vi "victory march sub vi (adjusted).vi"(11 "BrickReference in":T1) -> (3 "BrickReference out":T1)   [LabVIEW 2016]
uses:
  <vilib>/NXT/Subs/LVHSConnector.ctl
  <vilib>/NXT/LegoClasses/BrickReference/BrickReference.lvclass
  <vilib>/NXT/Dual Mode Library/Sound/PlayB.vi
  <vilib>/NXT/Dual Mode Library/Sound/PlayAsharp.vi
  <vilib>/NXT/Dual Mode Library/Sound/PlayC.vi
  <vilib>/NXT/Dual Mode Library/Sound/PlayD.vi
  <vilib>/NXT/Dual Mode Library/Sound/PlayE.vi
  <vilib>/NXT/Dual Mode Library/Sound/PlayG.vi
  <vilib>/NXT/Dual Mode Library/Sound/PlayFsharp.vi
  <vilib>/NXT/Dual Mode Library/Sound/PlayA.vi
  <vilib>/NXT/Dual Mode Library/Waits/Wait_Num.vi
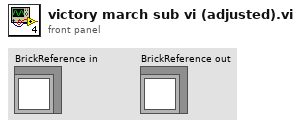
[diagram p1: front panel]
types:
  T1 = typedef "LVHSConnector.ctl" = refnum<class "BrickReference.lvclass">
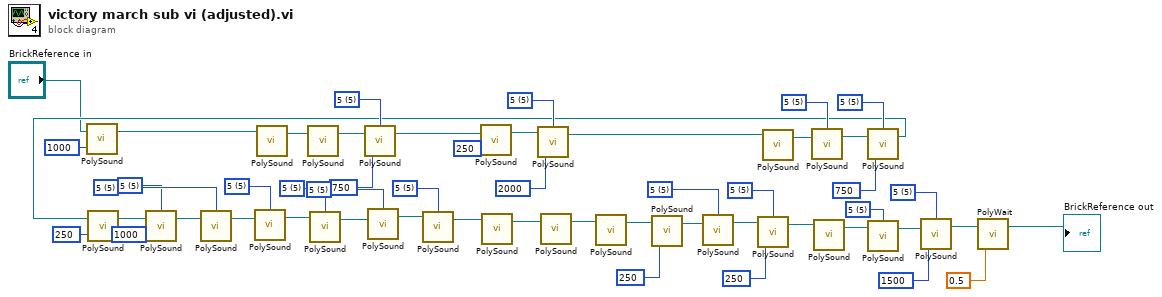
[diagram p0: block diagram]
diagram:
  w51 = u16 5 items=["3"=3, "4"=4, "5"=5, "6"=6, "7"=7] ("Octave")
  w50 = u16 5 items=["3"=3, "4"=4, "5"=5, "6"=6, "7"=7] ("Octave")
  w49 = u16 5 items=["3"=3, "4"=4, "5"=5, "6"=6, "7"=7] ("Octave")
  w48 = u16 5 items=["3"=3, "4"=4, "5"=5, "6"=6, "7"=7] ("Octave")
  w44 = u16 5 items=["3"=3, "4"=4, "5"=5, "6"=6, "7"=7] ("Octave")
  w43 = u16 5 items=["3"=3, "4"=4, "5"=5, "6"=6, "7"=7] ("Octave")
  w42 = u16 5 items=["3"=3, "4"=4, "5"=5, "6"=6, "7"=7] ("Octave")
  w41 = u16 5 items=["3"=3, "4"=4, "5"=5, "6"=6, "7"=7] ("Octave")
  w40 = u16 5 items=["3"=3, "4"=4, "5"=5, "6"=6, "7"=7] ("Octave")
  w36 = u16 5 items=["3"=3, "4"=4, "5"=5, "6"=6, "7"=7] ("Octave")
  w35 = u16 5 items=["3"=3, "4"=4, "5"=5, "6"=6, "7"=7] ("Octave")
  w34 = u16 5 items=["3"=3, "4"=4, "5"=5, "6"=6, "7"=7] ("Octave")
  w33 = u16 5 items=["3"=3, "4"=4, "5"=5, "6"=6, "7"=7] ("Octave")
  w32 = u16 5 items=["3"=3, "4"=4, "5"=5, "6"=6, "7"=7] ("Octave")
  n1 = call-poly <vilib>:"PolySound.vi"("Duration (500 ms)"=u16 1000, "NXT/EV3"="BrickReference in") -> ("NXT/EV3"=w5:T1)  [unwired: 2 in]
  n2 = call-poly <vilib>:"PolySound.vi"("NXT/EV3"=w5) -> ("NXT/EV3"=w6:T1)  [unwired: 3 in]
  n3 = call-poly <vilib>:"PolySound.vi"("NXT/EV3"=w6) -> ("NXT/EV3"=w7:T1)  [unwired: 3 in]
  n4 = call-poly <vilib>:"PolySound.vi"("Duration (500 ms)"=u16 750, "NXT/EV3"=w7, "Octave"=w32) -> ("NXT/EV3"=w4:T1)  [unwired: 1 in]
  n5 = call-poly <vilib>:"PolySound.vi"("Duration (500 ms)"=u16 250, "NXT/EV3"=w4) -> ("NXT/EV3"=w8:T1)  [unwired: 2 in]
  n6 = call-poly <vilib>:"PolySound.vi"("Duration (500 ms)"=u16 2000, "NXT/EV3"=w8, "Octave"=w33) -> ("NXT/EV3"=w3:T1)  [unwired: 1 in]
  n7 = call-poly <vilib>:"PolySound.vi"("NXT/EV3"=w3) -> ("NXT/EV3"=w9:T1)  [unwired: 3 in]
  n8 = call-poly <vilib>:"PolySound.vi"("NXT/EV3"=w9, "Octave"=w34) -> ("NXT/EV3"=w10:T1)  [unwired: 2 in]
  n9 = call-poly <vilib>:"PolySound.vi"("Duration (500 ms)"=u16 750, "NXT/EV3"=w10, "Octave"=w35) -> ("NXT/EV3"=w2:T1)  [unwired: 1 in]
  n10 = call-poly <vilib>:"PolySound.vi"("Duration (500 ms)"=u16 250, "NXT/EV3"=w2) -> ("NXT/EV3"=w11:T1)  [unwired: 2 in]
  n11 = call-poly <vilib>:"PolySound.vi"("Duration (500 ms)"=u16 1000, "NXT/EV3"=w11, "Octave"=w36) -> ("NXT/EV3"=w12:T1)  [unwired: 1 in]
  n12 = call-poly <vilib>:"PolySound.vi"("NXT/EV3"=w12, "Octave"=w40) -> ("NXT/EV3"=w13:T1)  [unwired: 2 in]
  n13 = call-poly <vilib>:"PolySound.vi"("NXT/EV3"=w13, "Octave"=w41) -> ("NXT/EV3"=w14:T1)  [unwired: 2 in]
  n14 = call-poly <vilib>:"PolySound.vi"("NXT/EV3"=w14, "Octave"=w42) -> ("NXT/EV3"=w15:T1)  [unwired: 2 in]
  n15 = call-poly <vilib>:"PolySound.vi"("NXT/EV3"=w15, "Octave"=w43) -> ("NXT/EV3"=w16:T1)  [unwired: 2 in]
  n16 = call-poly <vilib>:"PolySound.vi"("NXT/EV3"=w16, "Octave"=w44) -> ("NXT/EV3"=w17:T1)  [unwired: 2 in]
  n17 = call-poly <vilib>:"PolySound.vi"("NXT/EV3"=w17) -> ("NXT/EV3"=w18:T1)  [unwired: 3 in]
  n18 = call-poly <vilib>:"PolySound.vi"("NXT/EV3"=w18) -> ("NXT/EV3"=w19:T1)  [unwired: 3 in]
  n19 = call-poly <vilib>:"PolySound.vi"("NXT/EV3"=w19) -> ("NXT/EV3"=w20:T1)  [unwired: 3 in]
  n20 = call-poly <vilib>:"PolySound.vi"("Duration (500 ms)"=u16 250, "NXT/EV3"=w20) -> ("NXT/EV3"=w21:T1)  [unwired: 2 in]
  n21 = call-poly <vilib>:"PolySound.vi"("NXT/EV3"=w21, "Octave"=w48) -> ("NXT/EV3"=w22:T1)  [unwired: 2 in]
  n22 = call-poly <vilib>:"PolySound.vi"("Duration (500 ms)"=u16 250, "NXT/EV3"=w22, "Octave"=w49) -> ("NXT/EV3"=w23:T1)  [unwired: 1 in]
  n23 = call-poly <vilib>:"PolySound.vi"("NXT/EV3"=w23) -> ("NXT/EV3"=w24:T1)  [unwired: 3 in]
  n24 = call-poly <vilib>:"PolySound.vi"("NXT/EV3"=w24, "Octave"=w50) -> ("NXT/EV3"=w25:T1)  [unwired: 2 in]
  n25 = call-poly <vilib>:"PolySound.vi"("Duration (500 ms)"=u16 1500, "NXT/EV3"=w25, "Octave"=w51) -> ("NXT/EV3"=w26:T1)  [unwired: 1 in]
  n26 = call-poly <vilib>:"PolyWait.vi"("Time (1 sec)"=sgl 0.5, "NXT/EV3"=w26) -> ("NXT/EV3"=→"BrickReference out":T1)  [unwired: 2 in]
